vi "Build and Upload New Mission.vi"(8 "Error In":errorcluster) -> (0 "Error Out":errorcluster)   [LabVIEW 2014]
uses:
  Aircraft Information/Sub VI/Selected Aircraft/SubVI/Get Selected Aircraft.vi
  Aircraft Information/Sub VI/Set Aircraft Waypoints.vi
  Controls/MAVLINK Mav Frame.ctl
  Waypoint Controller/FGV/Methods/Set Waypoint Transfer Status.vi
  Waypoint Controller/Controls/Waypoint Transfer Status.ctl
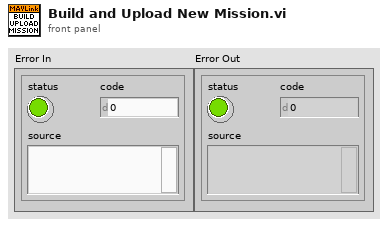
[diagram p1: front panel]
types:
  T1 = typedef "Waypoint Transfer Status.ctl" = cluster{"Upload Complete":bool, "Transfer Progress (Upload)":dbl, "Download Complete":bool, "Transfer Progress (Download)":dbl}
  T2 = typedef "MAVLINK Mav Frame.ctl" = enum8{"GLOBAL", "LOCAL NED", "MISSION", "GLOBAL RELATIVE ALT", "LOCAL ENU", "GLOBAL INT", "GLOBAL RELATIVE ALT INT", "LOCAL OFFSET NED", "BODY NED", "BODY OFFSET NED", "GLOBAL TERRAIN ALT", "GLOBAL TERRAIN ALT INT"}
  T3 = cluster{"target_system":u8, "target_component":u8, "sequence":u16, "frame":T2, "command":u16, "current":bool, "autocontinue":bool, "param1":sgl, "param2":sgl, "param3":sgl, "param4":sgl, "x":sgl, "y":sgl, "z":sgl}[]
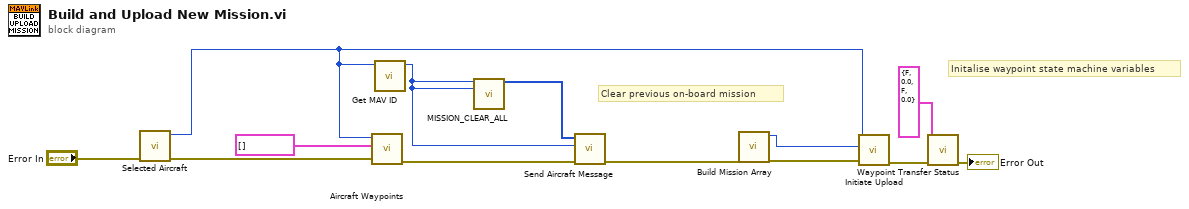
[diagram p0: block diagram]
diagram:
  # "Initalise waypoint state machine variables"
  # "Clear previous on-board mission"
  n1 = call-poly "Selected Aircraft.vi"("Error In"="Error In") -> ("Error Out"=w8:errorcluster, "Selected Aircraft ID Out"=w1:u8)  [unwired: 9 in]
  n2 = call-poly "Aircraft Waypoints.vi"("Error In"=w8, "Waypoints In"=T3 [], "Aircraft ID"=w1) -> ("Error Out"=w11:errorcluster)  [unwired: 8 in]
  n3 = call "Get MAV ID.vi"("Aircraft Index"=w1) -> ("Aircraft ID"=w10:u8)  [unwired: 9 in, 1 out]
  n4 = call "MISSION_CLEAR_ALL.vi"("target_system"=w10, "target_component"=w10) -> ("MAVLink Message"=w9:u8[])  [unwired: 13 in]
  n5 = call "Send Aircraft Message.vi"("error in (no error)"=w11, "Aircraft ID"=w10, "MAVLink Message"=w9) -> ("error out"=w6:errorcluster)  [unwired: 8 in]
  n6 = call "Build Mission Array.vi"("Error In"=w6) -> ("Error Out"=w12:errorcluster, "Number of Waypoints"=w13:i32)  [unwired: 9 in]
  n7 = call "Initiate Upload.vi"("Error In"=w12, "Number of Waypoints"=w13, "Aircraft Index"=w1) -> ("Error Out"=w5:errorcluster)  [unwired: 8 in]
  n8 = call-poly "Waypoint Transfer Status.vi"("Error In"=w5, "Waypoint Transfer Status In"=T1 {"Upload Complete"=FALSE, "Transfer Progress (Upload)"=0.0, "Download Complete"=FALSE, "Transfer Progress (Download)"=0.0}) -> ("Error Out"=→"Error Out":errorcluster)  [unwired: 9 in]
